vi "MAIN.vi"() -> ()   [LabVIEW 2020]
panel:
  out "d":dbl
  out "k":dbl
  out "y-Value":dbl
  out "XY Graph":cluster{"x-Wert":dbl[], "y-Wert":dbl[]}[](graph)
  out "Y1":dbl=3.5
  out "X1":dbl=0.5
  out "Y2":dbl=4.8
  in  "y-Wert":dbl[](array[numeric])=[1.0, 3.5, 4.8, 3.9, 2.7, 3.6, 4.1, 5.3]
  out "Index":i32=2
  out "X2":dbl=1.3
  in  "x-Value":dbl=1.2
  in  "x-Wert":dbl[](array[numeric])=[0.0, 0.5, 1.3, 1.9, 2.1, 2.5, 3.0, 3.3]
  # "Datenfeld x & y Werte"
  # "Interplation"
  # "Stützpunkte"
  # "Interpolationsgerade"
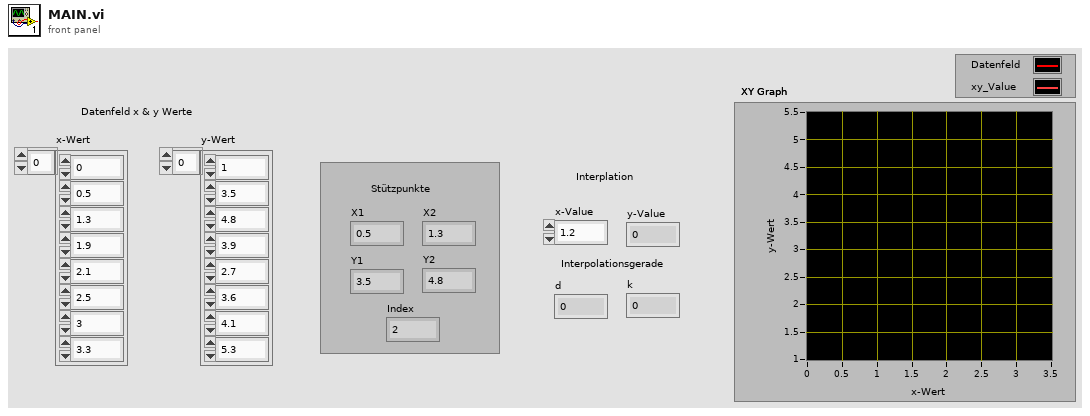
[diagram p1: front panel]
types:
  T1 = cluster{"Numeric 4":dbl, "Numeric 3":dbl, "Numeric 2":dbl, "Numeric":dbl}
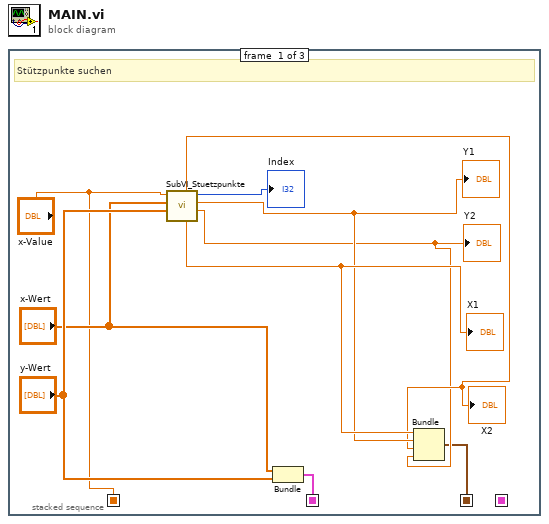
[diagram p0: block diagram]
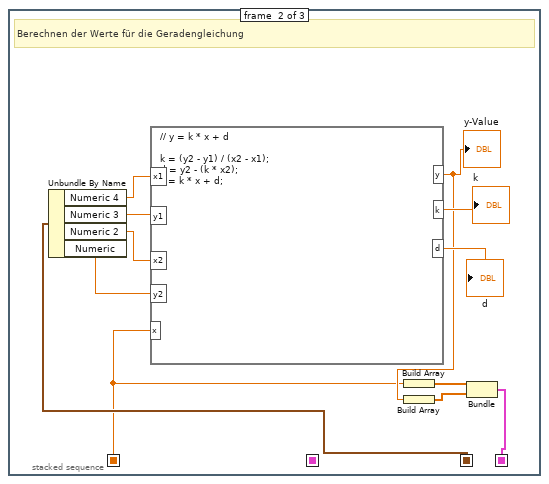
[diagram p2: hidden frame]
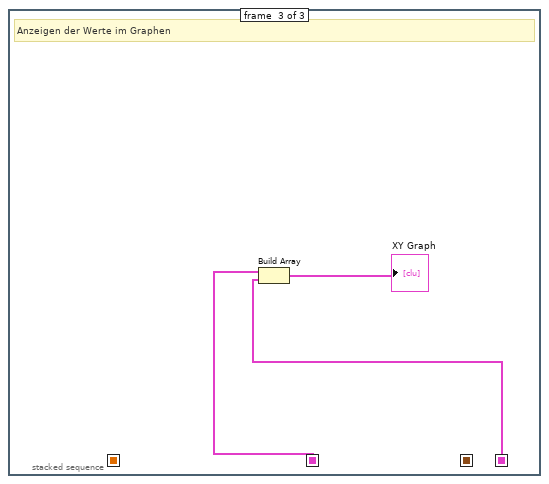
[diagram p3: hidden frame]
diagram:
  n1 = stacked-sequence {
    seq-local: [w8 _ _] -> [_ _ w25]
    seq-local: [w2 _ _] -> [_ w22 _]
    seq-local: ["x-Value" _ _] -> [_ w14 _]
    seq-local: [_ w11 _] -> [_ _ w24]
    frame #0 {
      # "Stützpunkte suchen"
      n2 = call "SubVI_Stuetzpunkte.vi"("y-Wert"="y-Wert", "x-Wert"="x-Wert", "x-Value"="x-Value") -> ("Numeric"=w3:dbl, "Numeric 3"=w5:dbl, "Index"=→"Index":i32, "Numeric 4"=w6:dbl, "Numeric 2"=w4:dbl)  [unwired: 3 in, 1 out]
      "X2" <- w4
      "Y2" <- w3
      "X1" <- w6
      "Y1" <- w5
      n3 = Bundle("x-Wert"="x-Wert", "y-Wert"="y-Wert") -> (w8:cluster{"x-Wert":dbl[], "y-Wert":dbl[]})  [unwired: 1 in]
      n4 = Bundle("Numeric 4"=w6, "Numeric 3"=w5, "Numeric 2"=w4, "Numeric"=w3) -> (w2:T1)  [unwired: 1 in]
    }
    frame #1 {
      # "Berechnen der Werte für die Geradengleichung"
      n5 = Unbundle By Name(w22) -> ("Numeric 4"=w21:dbl, "Numeric 3"=w20:dbl, "Numeric 2"=w19:dbl, "Numeric"=w18:dbl)
      n6 = formula code="// y = k * x + d\n\nk = (y2 - y1) / (x2 - x1);\nd = y2 - (k * x2);\ny = k * x + d;"("x1"=w21, "y1"=w20, "x2"=w19, "y2"=w18, "x"=w14) -> ("y"=w15:dbl, "k"=→"k":dbl, "d"=→"d":dbl)
      "y-Value" <- w15
      n7 = Build Array(w14) -> (w13:dbl[])
      n8 = Build Array(w15) -> (w12:dbl[])
      n9 = Bundle(w13, w12) -> (w11:cluster{dbl[], dbl[]})  [unwired: 1 in]
    }
    frame #2 {
      # "Anzeigen der Werte im Graphen"
      n10 = Build Array(w25, w24) -> (→"XY Graph":cluster{"x-Wert":dbl[], "y-Wert":dbl[]}[])
    }
  }
